vi "Create.vi"(8 "error in (no error)":errorcluster, 10 "ImagesFolder":path) -> (0 "error out":errorcluster, 3 "BoardDisplay out":refnum<class "BoardDisplay.lvclass">)   [LabVIEW 2015, in "TronviewPresentation.lvlib" / "BoardDisplay.lvclass"]
uses:
  BoardDisplay.lvclass
  BoardDisplay.lvclass/BoardDisplay.ctl
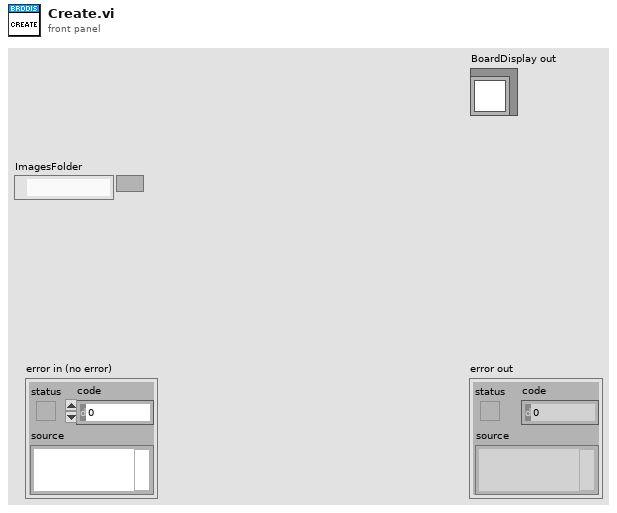
[diagram p1: front panel]
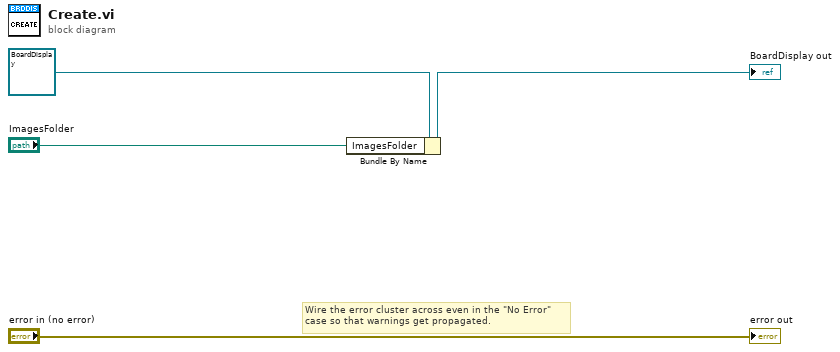
[diagram p0: block diagram]
diagram:
  # "Wire the error cluster across even in the \"No Error\"\ncase so that warnings get propagated."
  n1 = Bundle By Name(cluster=refnum<class "BoardDisplay.lvclass"> refnum ("BoardDisplay in"), "ImagesFolder"="ImagesFolder") -> (→"BoardDisplay out":refnum<class "BoardDisplay.lvclass">)
  "error out" <- "error in (no error)"
